vi "运维调试_CODCr.vi"() -> ()   [LabVIEW 2016, in "CODCr库.lvlib"]
uses:
  <vilib>/Utility/miscctls.llb/LVPointTypeDef.ctl
  <vilib>/ptbypt/NI_PtbyPt.lvlib
  <vilib>/Utility/config.llb/NI_LVConfig.lvlib
panel:
  in  "质控参数":bool
  in  "仪器参数":bool
  in  "MB通信方式选择":enum16{"串口", "TCP"}(ring)
  in  "释放串口":bool
  in  "打开串口":bool
  in  "加标回收测试":bool
  in  "平行样测试":bool
  in  "定时启动":bool
  out "COM口":string
  in  "空白测试":bool
  in  "隐藏按钮":bool
  in  "写入消解温度时长":bool
  in  "保存KB值":bool
  in  "标样核查":bool
  out "启动时间":timestamp format="%<%Y/%m/%d %H:%M:%S>T"
  out "主循环次数":i32
  out "status":bool
  out "启动测量模式":T1(ring)
  out "曲线截距B":sgl format="%#_10g"
  out "曲线斜率K":sgl format="%#_10g"
  out "量程上限":sgl
  out "量程下限":sgl
  out "消解时长":u16
  out "消解温度":u16
  out "测量精度":u16
  out "测量结果":sgl
  out "标样参考值":sgl
  out "量程":u16
  out "工作状态":T1(ring)
  out "仪器时间":timestamp format="%<%X\n%x>T"
  out "关键参数区":T2
  out "状态告警区":T3 {"告警代码" items=["无告警", "缺试剂告警", "缺水样告警", "缺蒸馏水告警", "缺标液告警", "仪表漏液告警", "标定异常告警", "超量程告警", "加热异常", "低试剂预警", "超上限告警", "超下限告警", "仪表内部其他异常", "滴定异常告警", "电极异常告警", "量程切换告警", "参数设置告警", "PH电极电位异常", "电导率电极异常", "浊度光度异常", "溶解氧电极异常", "溶解氧光强异常", "温度异常告警", "PH异常告警", "溶解氧异常告警", "电导率异常告警", "浊度异常告警", "叶绿素异常告警", "藻密度异常告警", "蓝绿藻异常告警", "ORP异常告警", "氨氮异常告警", "清洁刷异常告警", "SD卡异常告警", "蓝牙异常告警", "Wifi异常告警", "流程异常告警"]; "故障代码" items=["无故障", "电机故障", "温度故障", "通讯故障", "滴定故障"]}
  out "测量数据区":T4 {"单位" items=["ug/L", "mg/L", "ppm", "mg/m3", "cm", "ppb", "ug/m3", "%", "nmol/mol", "umol/mol", "MPN/L", "MPN/100ml", "ng/m3", "NTU", "无量纲", "ms/cm", "us/cm", "℃", "mV", "万个/L"]}
  out "系统时间":timestamp format="%<%Y/%m/%d %H:%M:%S>T"
  in  "停止":bool
  in  "校时":bool
  in  "标样校准":bool
  in  "空白校准":bool
  in  "零点核查":bool
  in  "跨度核查":bool
  in  "水样测试":bool
  in  "返回":bool
  in  "设置":bool
  # "mg/L"
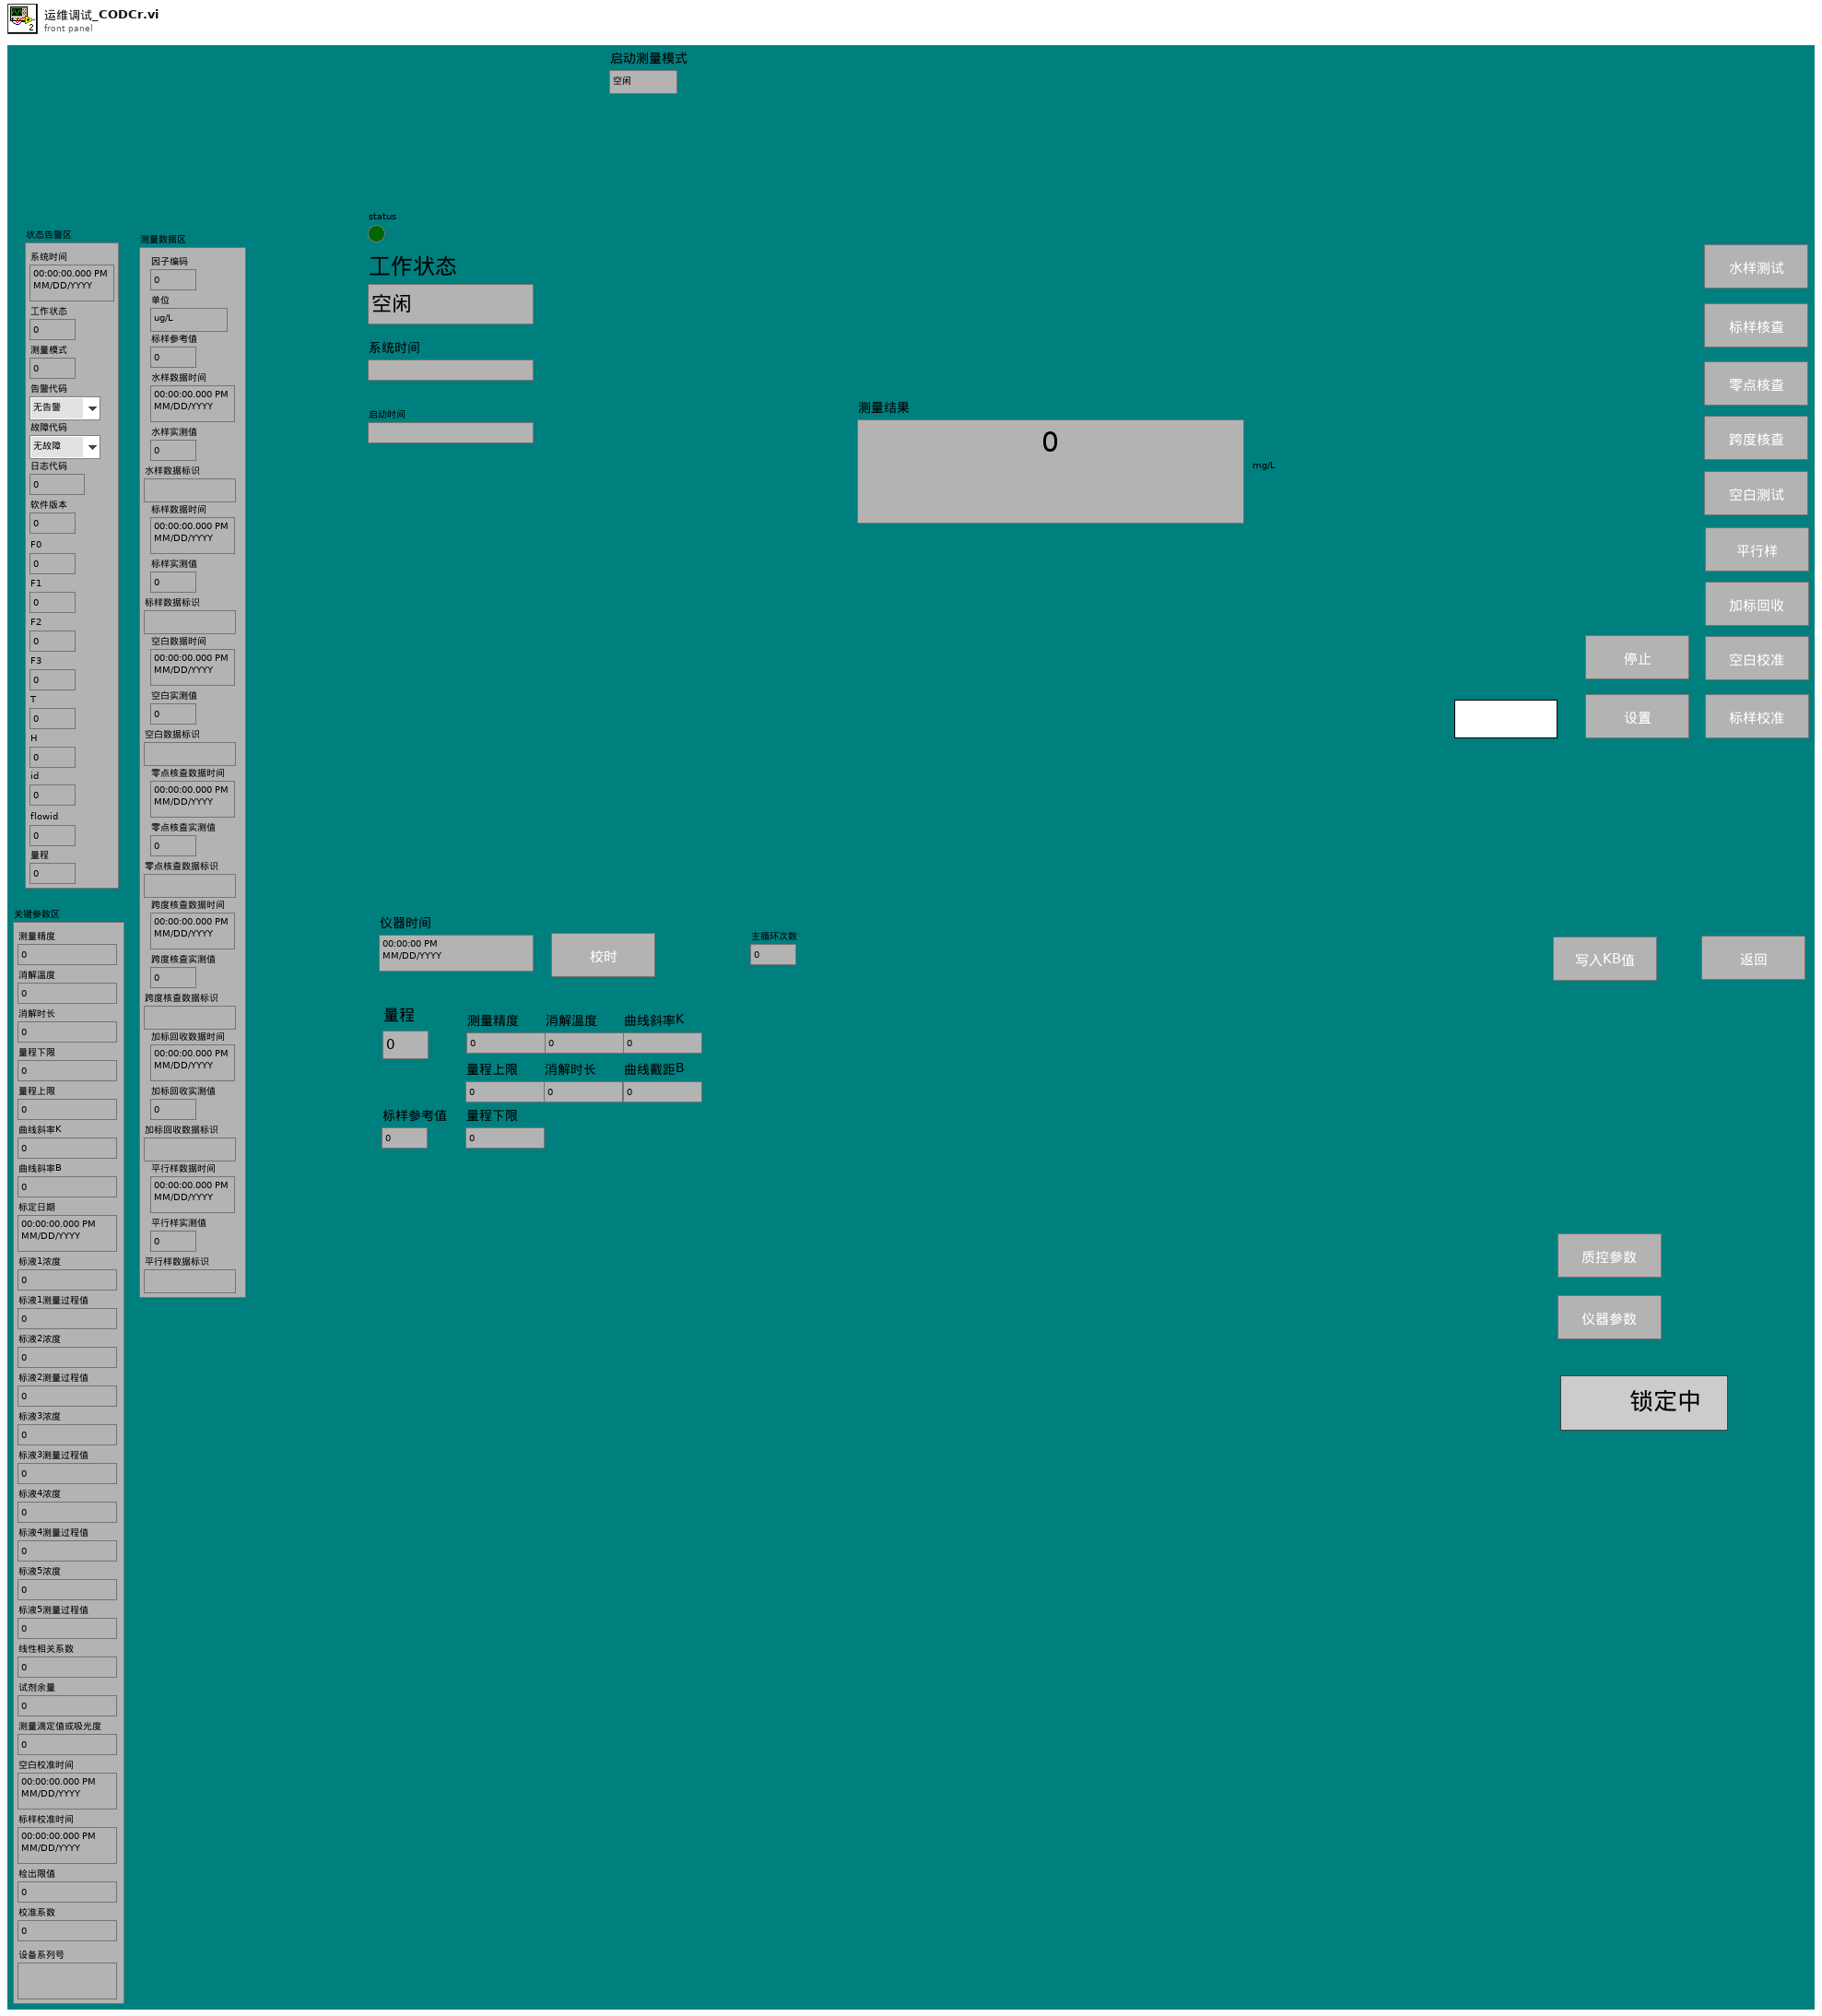
[diagram p1: front panel]
types:
  T1 = enum16{"空闲", "水样测试", "标样核查", "零点核查", "跨度核查", "空白测试", "平行样测试", "加标回收", "空白校准", "标样校准", "初始化（清洗）"}
  T2 = cluster{"测量精度":u16, "消解温度":u16, "消解时长":u16, "量程下限":sgl, "量程上限":sgl, "曲线斜率K":sgl, "曲线斜率B":sgl, "标定日期":timestamp, "标液1浓度":sgl, "标液1测量过程值":sgl, "标液2浓度":sgl, "标液2测量过程值":sgl, "标液3浓度":sgl, "标液3测量过程值":sgl, "标液4浓度":sgl, "标液4测量过程值":sgl, "标液5浓度":sgl, "标液5测量过程值":sgl, "线性相关系数":sgl, "试剂余量":u32, "测量滴定值或吸光度":sgl, "空白校准时间":timestamp, "标样校准时间":timestamp, "检出限值":sgl, "校准系数":sgl, "设备系列号":string}
  T3 = cluster{"系统时间":timestamp, "工作状态":u16, "测量模式":u16, "告警代码":u16, "故障代码":u16, "日志代码":u16, "软件版本":u16, "F0":sgl, "F1":sgl, "F2":sgl, "F3":sgl, "T":sgl, "H":sgl, "id":u16, "flowid":u16, "量程":u16}
  T4 = cluster{"因子编码":u32, "单位":u16, "标样参考值":sgl, "水样数据时间":timestamp, "水样实测值":sgl, "水样数据标识":string, "标样数据时间":timestamp, "标样实测值":sgl, "标样数据标识":string, "空白数据时间":timestamp, "空白实测值":sgl, "空白数据标识":string, "零点核查数据时间":timestamp, "零点核查实测值":sgl, "零点核查数据标识":string, "跨度核查数据时间":timestamp, "跨度核查实测值":sgl, "跨度核查数据标识":string, "加标回收数据时间":timestamp, "加标回收实测值":sgl, "加标回收数据标识":string, "平行样数据时间":timestamp, "平行样实测值":sgl, "平行样数据标识":string}
  T5 = cluster{"命令":string, "测量模式":enum16{"水样测量", "标样核查", "零点核查", "跨度核查", "空白测试", "加标回收", "平行样", "校零", "校标"}, "CODCr量程切换":enum32{"H", "L", "AUTO"}}
  T6 = typedef "LVPointTypeDef.ctl" = cluster{"Horizontal":i16, "Vertical":i16}
  T7 = typedef "NI_LVConfig.lvlib/Config Data RefNum.ctl" = refnum<k1>
  T8 = cluster{"运行模式":enum16{"维护模式", "常规模式", "应急模式", "质控模式"}}
  T9 = cluster{"时间标识":timestamp, "监测值":sgl, "单位":u16, "数据标识":string, "因子编码":u32, "标样参考值":sgl, "F0":sgl, "F1":sgl, "F2":sgl, "F3":sgl, "温度":sgl, "湿度":sgl, "量程标识":string, "LastTime":timestamp}
  T10 = cluster{"时间标识":timestamp, "设备":string, "日志信息":string}
  T11 = cluster{"时间标识":timestamp, "参数":string, "日志信息":string, "流程参数":string}
  T12 = cluster{"时间标识":timestamp, "设备":string, "日志信息":string, "流程参数":string}
  T13 = enum16{"水样测量", "标样核查", "零点核查", "跨度核查", "空白测试", "加标回收", "平行样", "校零", "校标"}
  T14 = cluster{"控制命令":enum16{"启动测量", "标样核查", "零点核查", "跨度核查", "空白测试", "平行样测试", "加标回收", "空白校准", "标样校准", "初始化（清洗）", "停止测试", "仪器重启", "校时", "模式设置", "测量间隔设置"}, "周期设置类型":enum16{"定点启动", "间隔启动"}, "定时功能启用":bool, "定时间隔":dbl, "24H周期设置":bool[], "零点核查时间":u16, "跨度核查时间":u16, "质控频次":enum16{"关闭", "每天", "星期一", "星期二", "星期三", "星期四", "星期五", "星期六", "星期日"}}
  T15 = cluster{"测量量程":dbl, "测量精度":dbl, "测量间隔":dbl, "消解温度":dbl, "消解时长":dbl, "空白校准时间":timestamp, "曲线截距":dbl, "曲线斜率":dbl, "测量检出限":dbl, "测量信号值":dbl, "线性相关系数":dbl, "二次多项式系数":dbl, "标样校准时间":timestamp, "稀释倍数":dbl, "三项式系数":dbl, "空白标定系数":dbl, "量程系数":dbl, "F0/ORPA":dbl, "F1/ORPB":dbl, "F2/ORPK":dbl, "F3":dbl, "F4":dbl, "F5":dbl, "F6":dbl, "F7":dbl, "X0/滴定数":dbl, "量程":dbl}
  T16 = cluster{"控制命令":enum16{"启动测量", "标样核查", "零点核查", "跨度核查", "空白测试", "平行样测试", "加标回收", "空白校准", "标样校准", "初始化（清洗）", "停止测试", "仪器重启", "校时", "模式设置", "测量间隔设置"}, "周期设置类型":enum16{"定点启动", "间隔启动"}, "定时功能启用":bool, "定时间隔":dbl, "24H周期设置":bool[], "空白核查时间":u16, "跨度核查时间":u16, "质控频次":enum16{"关闭", "每天", "星期一", "星期二", "星期三", "星期四", "星期五", "星期六", "星期日"}}
  T17 = cluster{"确定":bool, "测量量程":dbl, "测量精度":dbl, "测量间隔":dbl, "消解温度":dbl, "消解时长":dbl, "空白校准时间":timestamp, "曲线截距":dbl, "曲线斜率":dbl, "测量检出限":dbl, "测量信号值":dbl, "线性相关系数":dbl, "二次多项式系数":dbl, "标样校准时间":timestamp, "稀释倍数":dbl, "三项式系数":dbl, "空白标定系数":dbl, "量程系数":dbl, "F0/ORPA":dbl, "F1/ORPB":dbl, "F2/ORPK":dbl, "F3":dbl, "F4":dbl, "F5":dbl, "F6":dbl, "F7":dbl, "X0/滴定数":dbl, "量程":dbl}
  T18 = cluster{"跨度值":dbl, "零点标准液浓度":dbl, "跨度标准液浓度":dbl, "标准液标准浓度":dbl}
  T19 = cluster{"确定":bool, "跨度值":dbl, "零点标准液浓度":dbl, "跨度标准液浓度":dbl, "标准液标准浓度":dbl}
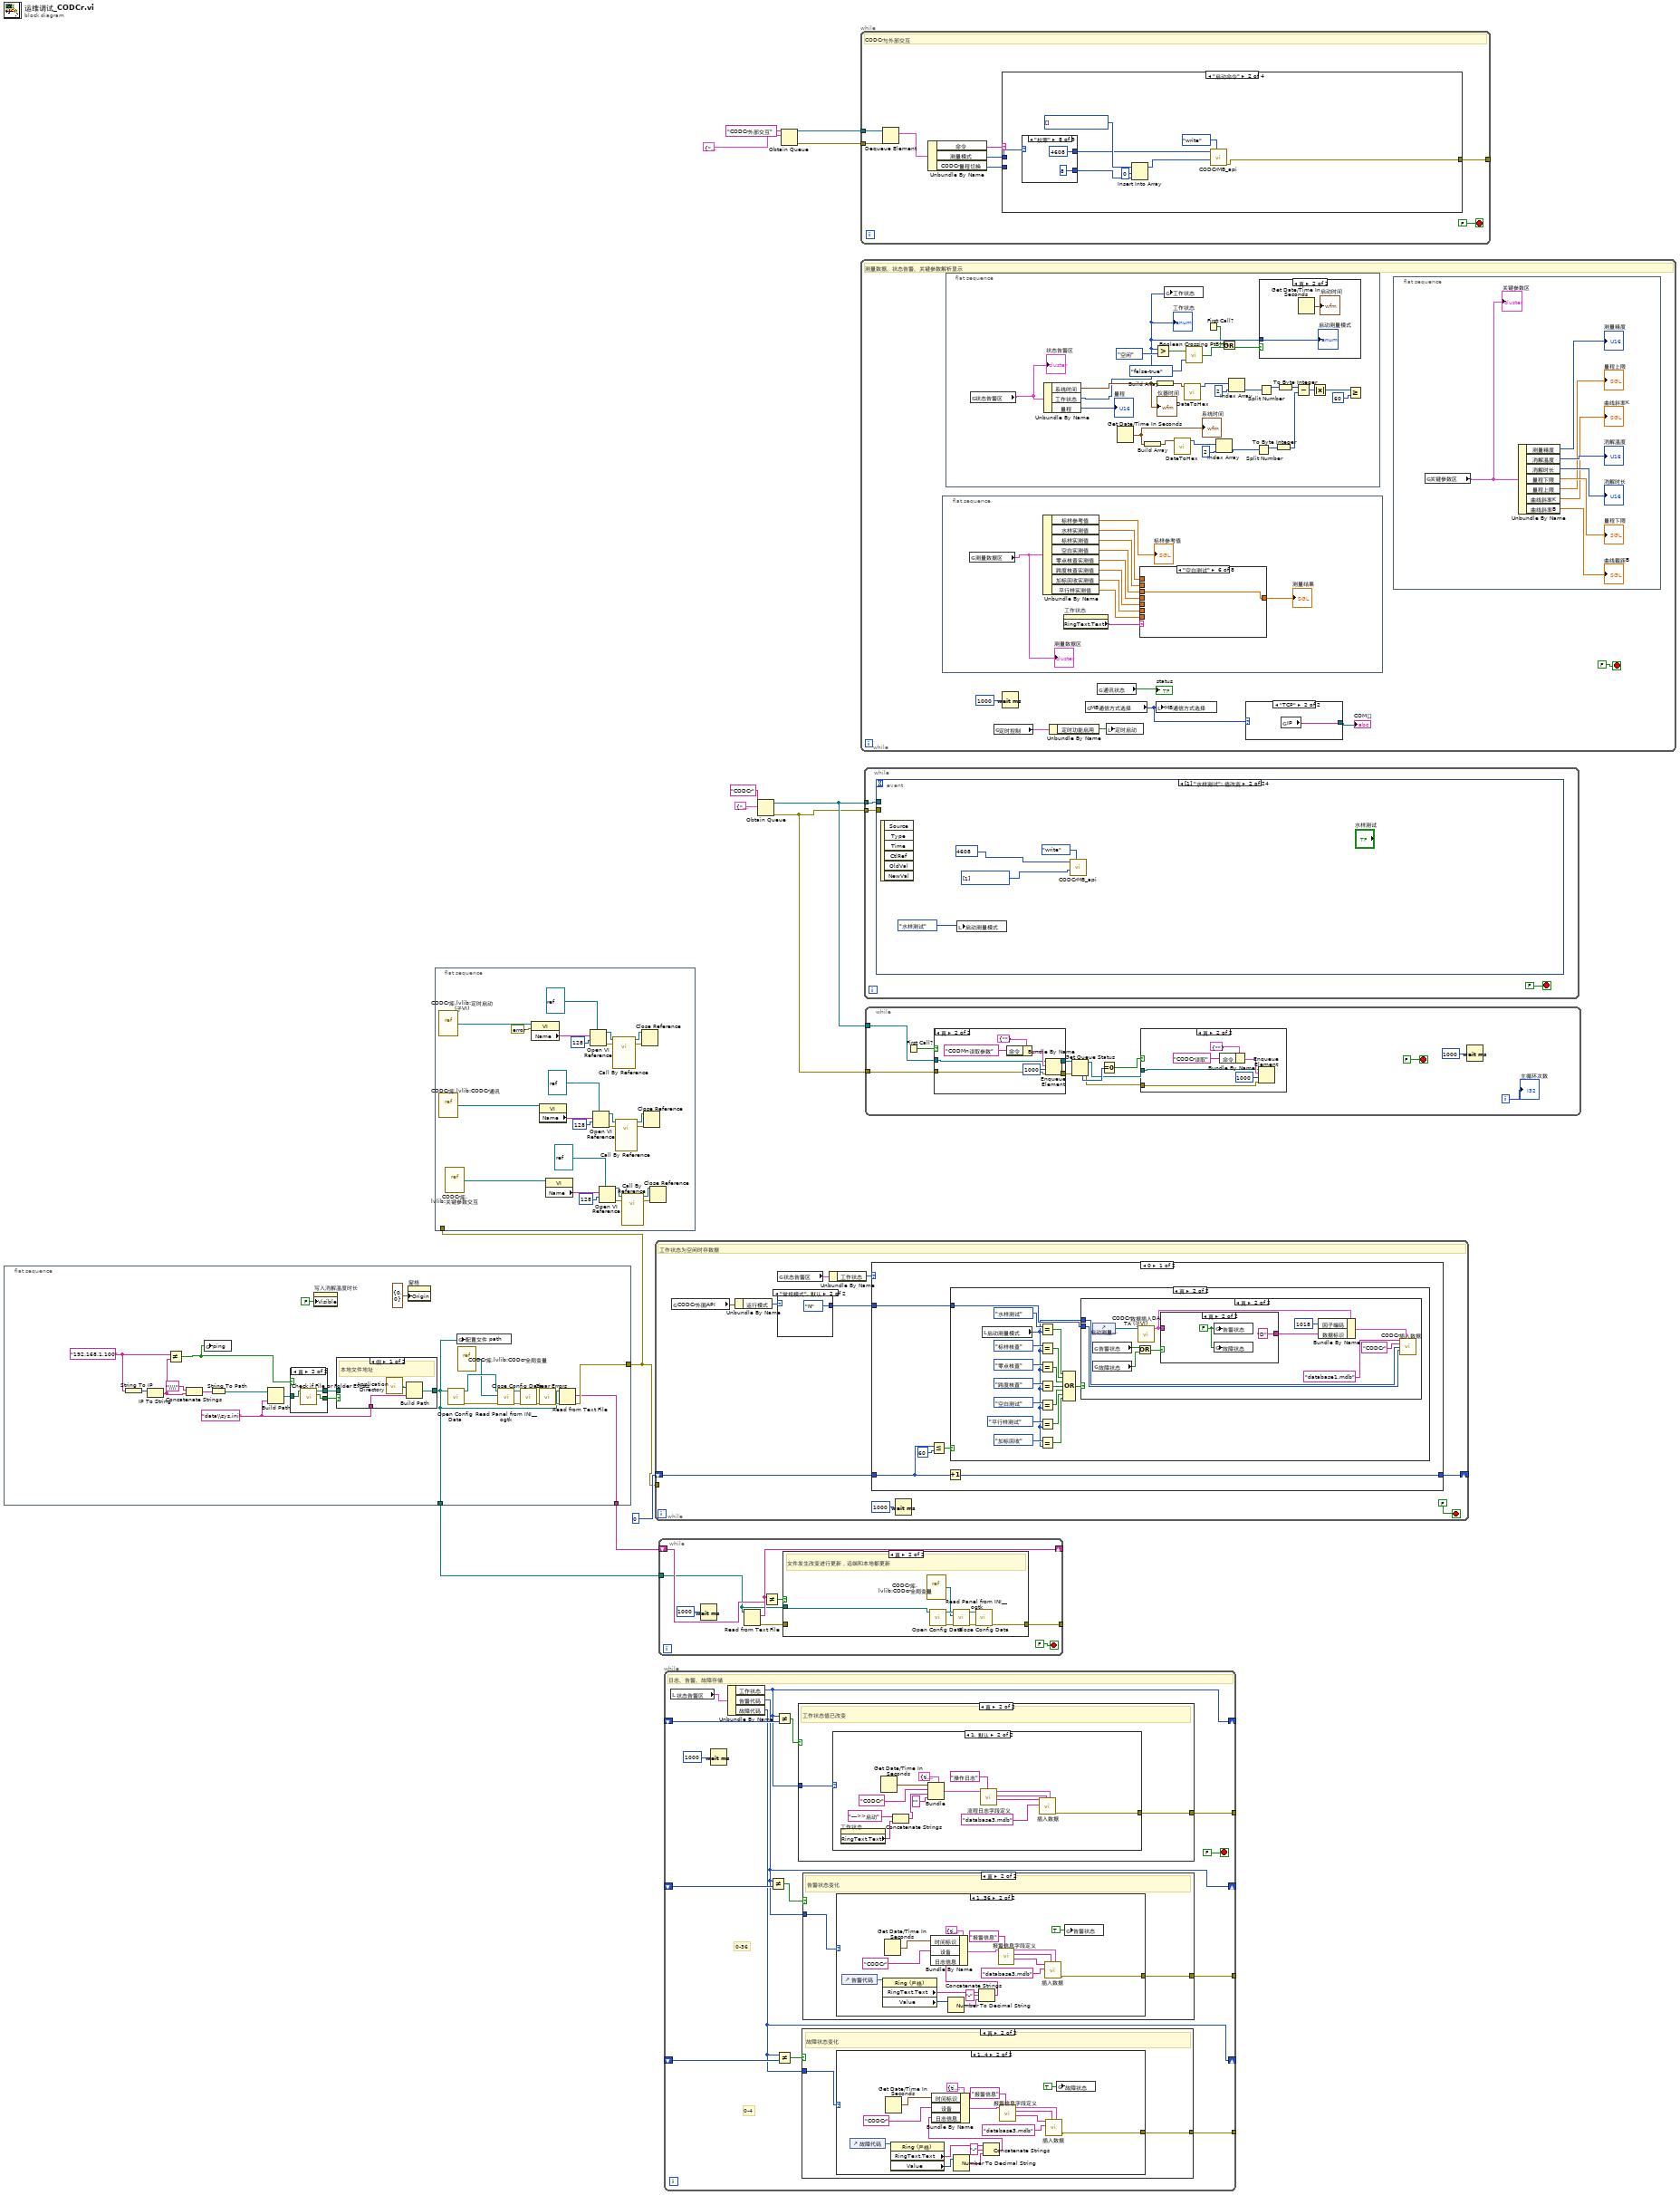
[diagram p0: block diagram]
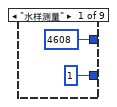
[diagram p6: hidden frame]
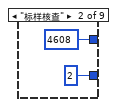
[diagram p7: hidden frame]
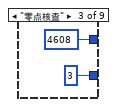
[diagram p8: hidden frame]
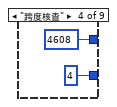
[diagram p9: hidden frame]
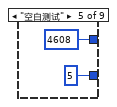
[diagram p10: hidden frame]
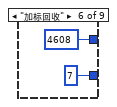
[diagram p11: hidden frame]
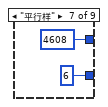
[diagram p12: hidden frame]
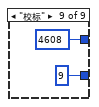
[diagram p13: hidden frame]
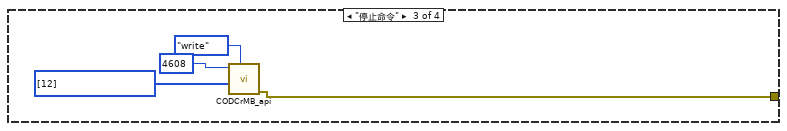
[diagram p14: hidden frame]
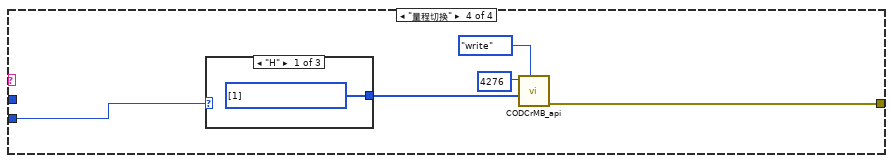
[diagram p15: hidden frame]
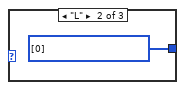
[diagram p16: hidden frame]
diagram:
  n1 = flat-sequence {
    tunnel: [w15] -> w1
    tunnel: [w14] -> w3
    tunnel: [w13] -> w2
    frame #0 {
      w33 = "data\\sys.ini" ("名称或相对路径")
      w18 = "192.168.1.100" ("名称")
      n2 = String To IP(1:w18) -> (0:w25:u32)
      n3 = IP To String(2:w25) -> (0:w22:string)  [unwired: 1 in]
      n4 = Not Equal?(x=w18, y=w22) -> (x != y?=w32:bool)
      n5 = Concatenate Strings("\\\\" ("字符串"), w22) -> (w23:string)
      n6 = global write "CODcr全局变量.vi" "ping"(w32) -> ()
      n7 = String To Path(string=w23) -> (path=w17:path)
      n8 = Build Path(base path=w17, name or relative path=w33) -> (appended path=w21:path)
      n9 = case shown="真" w32 {
        tunnel: w21 -> [w36 w40]
        tunnel: [w36 w39] -> w20
        tunnel: [FALSE w38] -> w19
        frame False {
        }
        frame True {
          n10 = call <vilib>:"Check if File or Folder Exists.vi"("path"=w40) -> ("file or folder exists?"=w38:bool, "dup path"=w39:path)  [unwired: 8 in, 1 out]
        }
      }
      n11 = property on="写入消解温度时长" class="Bool"("Visible"=FALSE ("可见")) -> ()  [unwired: 2 in, 2 out]
      n12 = case shown="假" w19 {
        tunnel: w20 -> [_ w44]
        tunnel: [w42 w44] -> w13
        tunnel: w33 -> [w41 _]
        frame False {
          # "本地文件地址"
          n13 = call <vilib>:"Application Directory.vi"() -> ("Application Directory"=w43:path)
          n14 = Build Path(base path=w43, name or relative path=w41) -> (appended path=w42:path)
        }
        frame True {
          # "网络共享地址"
        }
      }
      n15 = property on="窗格" class="Pane"("Origin"=T6 {"Horizontal"=0, "Vertical"=0} ("原点")) -> ()  [unwired: 2 in, 2 out]
      n16 = call <vilib>:"Open Config Data.vi"("configuration file path"=w13) -> ("error out"=w29:errorcluster, "refnum"=w28:T7)  [unwired: 8 in, 1 out]
      n17 = global write "CODcr全局变量.vi" "配置文件 path"(w13) -> ()
      n18 = vi-ref "CODCr库.lvlib:CODcr全局变量.vi"() -> (w16:refnum<vi>)
      n19 = call <userlib>:"Read Panel from INI__ogtk.vi"("error in (no error)"=w29, "VI ref"=w16, "refnum"=w28) -> ("error out"=w27:errorcluster, "refnum out"=w26:T7)  [unwired: 7 in]
      n20 = call <vilib>:"Close Config Data.vi"("error in (no error)"=w27, "refnum"=w26) -> ("error out"=w30:errorcluster)  [unwired: 8 in, 1 out]
      n21 = call <vilib>:"Clear Errors.vi"("error in (no error)"=w30) -> ("error out"=w31:errorcluster)  [unwired: 5 in, 1 out]
      n22 = Read from Text File(file (use dialog)=w13, error in=w31) -> (text=w14:string, error out=w15:errorcluster)  [unwired: 2 in, 2 out]
    }
  }
  n23 = flat-sequence {
    tunnel: w1 -> [_]
    frame #0 {
      n24 = vi-ref "CODCr库.lvlib:定时启动 (子VI).vi"() -> (w53:refnum<vi>)
      n25 = vi-ref "CODCr库.lvlib:CODCr通讯.vi"() -> (w62:refnum<vi>)
      n26 = vi-ref "CODCr库.lvlib:关键参数交互.vi"() -> (w52:refnum<vi>)
      n27 = property class="VI"(reference=w53, error in=errorcluster {"status"=FALSE, "code"=0, "source"=""} ("错误输出")) -> ("Name"=w54:string)  [unwired: 2 out]
      n28 = property class="VI"(reference=w62) -> ("Name"=w63:string)  [unwired: 1 in, 2 out]
      n29 = property class="VI"(reference=w52) -> ("Name"=w51:string)  [unwired: 1 in, 2 out]
      n30 = Open VI Reference(type specifier VI Refnum (for type only)=refnum<vi> refnum, vi path=w54, options=128 ("选项")) -> (vi reference=w56:refnum<vi>, error out=w58:errorcluster)  [unwired: 3 in]
      n31 = Open VI Reference(type specifier VI Refnum (for type only)=refnum<vi> refnum, vi path=w63, options=128 ("选项")) -> (vi reference=w65:refnum<vi>, error out=w67:errorcluster)  [unwired: 3 in]
      n32 = Open VI Reference(type specifier VI Refnum (for type only)=refnum<vi> refnum, vi path=w51, options=128 ("选项")) -> (vi reference=w49:refnum<vi>, error out=w47:errorcluster)  [unwired: 3 in]
      n33 = call-by-ref "?"(reference=w56, error in=w58) -> (reference out=w60:refnum<vi>, error out=w59:errorcluster)  [unwired: 12 in]
      n34 = call-by-ref "?"(reference=w65, error in=w67) -> (reference out=w69:refnum<vi>, error out=w68:errorcluster)  [unwired: 12 in]
      n35 = call-by-ref "?"(reference=w49, error in=w47) -> (reference out=w45:refnum<vi>, error out=w46:errorcluster)  [unwired: 12 in]
      n36 = Close Reference(reference=w60, error in (no error)=w59) -> ()  [unwired: 1 out]
      n37 = Close Reference(reference=w69, error in (no error)=w68) -> ()  [unwired: 1 out]
      n38 = Close Reference(reference=w45, error in (no error)=w46) -> ()  [unwired: 1 out]
    }
  }
  n39 = while "While循环" {
    tunnel: w1 -> [_]
    shift-right: [w70] -> _
    shift-left: 0 -> [w71]
    stop <- FALSE stop-if-true
    # "工作状态为空闲时存数据"
    n40 = global read "CODCr外部API.vi" "CODCr外围API"() -> (w74:T8)
    n41 = Unbundle By Name(w74) -> ("运行模式"=w73:enum16{"维护模式", "常规模式", "应急模式", "质控模式"})
    n42 = global read "CODcr全局变量.vi" "状态告警区"() -> (w72:T3)
    n43 = case shown="\"常规模式\", 默认" w73 {
      tunnel: [enum16{"N", "M"}."M" ("数据类型") enum16{"N", "M"}."N" ("数据类型")] -> w75
      frame "维护模式" {
      }
      frame "常规模式", Default {
      }
    }
    n44 = Unbundle By Name(w72) -> ("工作状态"=w76:u16)
    n45 = case shown="0" w76 {
      tunnel: w75 -> [w85 _]
      tunnel: w71 -> [w83 _]
      tunnel: [w84 _] -> w70
      frame 0 {
        n46 = Less Or Equal?(x=w83, y=60) -> (x <= y?=w81:bool)
        n47 = Increment(x=w83) -> (x+1=w84:i32)
        n48 = case shown="真" w81 {
          tunnel: w85 -> [_ w102]
          frame False {
          }
          frame True {
            n49 = local read "启动测量模式"() -> (w94:T1)
            n50 = Equal?(x=T1."水样测试" ("启动测量模式"), y=w94) -> (x = y?=w93:bool)
            n51 = Equal?(x=T1."标样核查" ("启动测量模式"), y=w94) -> (x = y?=w92:bool)
            n52 = Equal?(x=T1."零点核查" ("启动测量模式"), y=w94) -> (x = y?=w91:bool)
            n53 = Equal?(x=T1."跨度核查" ("启动测量模式"), y=w94) -> (x = y?=w90:bool)
            n54 = Equal?(x=T1."空白测试" ("启动测量模式"), y=w94) -> (x = y?=w89:bool)
            n55 = Equal?(x=T1."平行样测试" ("启动测量模式"), y=w94) -> (x = y?=w88:bool)
            n56 = Equal?(x=T1."加标回收" ("启动测量模式"), y=w94) -> (x = y?=w87:bool)
            n57 = Compound Arithmetic op=OR(w93, w92, w91, w90, w89, w88, w87) -> (w86:bool)
            n58 = case shown="真" w86 {
              tunnel: w94 -> [_ w110]
              tunnel: w102 -> [_ w109]
              frame False {
              }
              frame True {
                n59 = control-ref of="启动测量模式"() -> (w114:refnum<vi>)
                n60 = global read "CODcr全局变量.vi" "告警状态"() -> (w107:bool)
                n61 = global read "CODcr全局变量.vi" "故障状态"() -> (w106:bool)
                n62 = Or(x=w107, y=w106) -> (x .or. y?=w105:bool)
                n63 = call "CODCr数据插入DATA (子VI).vi"("Enum输入"=w114) -> ("data"=w104:T9)  [unwired: 10 in]
                n64 = case shown="真" w105 {
                  tunnel: w104 -> [w116 _]
                  tunnel: [w115 "D" ("table")] -> w103
                  frame False {
                    n65 = Unbundle By Name(w116) -> ("数据标识"=w115:string)
                  }
                  frame True {
                    w117 = FALSE ("告警状态")
                    n66 = global write "CODcr全局变量.vi" "告警状态"(w117) -> ()
                    n67 = global write "CODcr全局变量.vi" "故障状态"(w117) -> ()
                  }
                }
                n68 = Bundle By Name(cluster=w104, "因子编码"=u32 1018, "数据标识"=w103) -> (w113:T9)
                n69 = call "CODCr插入数据.vi"("database"="database1.mdb", "data"=w113, "table"="CODCr", "测量模式"=w110, "数据类型"=w109) -> ()  [unwired: 10 in, 1 out]
              }
            }
          }
        }
      }
      frame 1, Default {
      }
    }
    n70 = Wait (ms)(milliseconds to wait=u32 1000 ("等待时间（毫秒）")) -> ()  [unwired: 1 out]
  }
  n71 = while {
    tunnel: [w125] -> _
    shift-right: [w123] -> _
    shift-left: w3 -> [w122]
    tunnel: w2 -> [w119]
    stop <- FALSE stop-if-true
    n72 = Wait (ms)(milliseconds to wait=u32 1000 ("等待时间（毫秒）")) -> ()  [unwired: 1 out]
    n73 = Read from Text File(file (use dialog)=w119) -> (text=w123:string, error out=w120:errorcluster)  [unwired: 3 in, 2 out]
    n74 = Not Equal?(x=w123, y=w122) -> (x != y?=w121:bool)
    n75 = case shown="真" w121 {
      tunnel: [w127 w134] -> w125
      tunnel: w119 -> [_ w128]
      tunnel: w120 -> [w127 _]
      frame False {
      }
      frame True {
        # "文件发生改变进行更新，远端和本地都更新"
        n76 = vi-ref "CODCr库.lvlib:CODcr全局变量.vi"() -> (w129:refnum<vi>)
        n77 = call <vilib>:"Open Config Data.vi"("configuration file path"=w128) -> ("error out"=w133:errorcluster, "refnum"=w132:T7)  [unwired: 8 in, 1 out]
        n78 = call <userlib>:"Read Panel from INI__ogtk.vi"("error in (no error)"=w133, "VI ref"=w129, "refnum"=w132) -> ("error out"=w131:errorcluster, "refnum out"=w130:T7)  [unwired: 7 in]
        n79 = call <vilib>:"Close Config Data.vi"("error in (no error)"=w131, "refnum"=w130) -> ("error out"=w134:errorcluster)  [unwired: 8 in, 1 out]
      }
    }
  }
  n80 = while {
    shift-right: [w145] -> _
    shift-left: _ -> [w147]
    tunnel: [w144] -> _
    shift-right: [w141] -> _
    shift-left: _ -> [w142]
    shift-right: [w137] -> _
    shift-left: _ -> [w139]
    tunnel: [w138] -> _
    tunnel: [w136] -> _
    stop <- FALSE stop-if-true
    # "0-4"
    # "0-36"
    # "日志、告警、故障存储"
    n81 = local read "状态告警区"() -> (w135:T3)
    n82 = Wait (ms)(milliseconds to wait=u32 1000 ("等待时间（毫秒）")) -> ()  [unwired: 1 out]
    n83 = Unbundle By Name(w135) -> ("工作状态"=w145:u16, "告警代码"=w141:u16, "故障代码"=w137:u16)
    n84 = Not Equal?(x=w141, y=w142) -> (x != y?=w143:bool)
    n85 = Not Equal?(x=w145, y=w147) -> (x != y?=w146:bool)
    n86 = Not Equal?(x=w137, y=w139) -> (x != y?=w140:bool)
    n87 = case shown="真" w146 {
      tunnel: w145 -> [_ w189]
      tunnel: [_ w188] -> w144
      frame False {
      }
      frame True {
        # "工作状态值已改变"
        n88 = case shown="1, 默认" w189 {
          tunnel: [w190 w205] -> w188
          frame 0 {
            n89 = Get Date/Time In Seconds() -> (seconds since 1Jan1904=w197:timestamp)
            n90 = Bundle(cluster=T11 {"时间标识"=timestamp(0 s since 1904-01-01), "参数"="", "日志信息"="", "流程参数"=""} ("data in"), "时间标识"=w197, "参数"="CODCr" ("table输入"), "日志信息"="--->>结束", "流程参数"="" ("table输入")) -> (w191:T11)
            n91 = call "流程日志字段定义.vi"("table输入"="操作日志", "data in"=w191) -> ("table输出"=w195:string, "columns"=w193:string[], "data out"=w192:T12)  [unwired: 7 in]
            n92 = call "插入数据.vi"("data"=w192, "columns"=w193, "database"="database3.mdb", "table"=w195) -> ("error out"=w190:errorcluster)  [unwired: 7 in]
          }
          frame 1, Default {
            n93 = property on="工作状态" class="Enum (严格)"() -> ("RingText.Text"=w202:string)  [unwired: 2 in, 2 out]
            n94 = Get Date/Time In Seconds() -> (seconds since 1Jan1904=w212:timestamp)
            n95 = Concatenate Strings("--->>启动" ("日志信息"), w202) -> (w203:string)
            n96 = Bundle(cluster=T11 {"时间标识"=timestamp(0 s since 1904-01-01), "参数"="", "日志信息"="", "流程参数"=""} ("data in"), "时间标识"=w212, "参数"="CODCr" ("table输入"), "日志信息"=w203, "流程参数"="" ("table输入")) -> (w211:T11)
            n97 = call "流程日志字段定义.vi"("table输入"="操作日志", "data in"=w211) -> ("table输出"=w209:string, "columns"=w207:string[], "data out"=w206:T12)  [unwired: 7 in]
            n98 = call "插入数据.vi"("data"=w206, "columns"=w207, "database"="database3.mdb", "table"=w209) -> ("error out"=w205:errorcluster)  [unwired: 7 in]
          }
        }
      }
    }
    n99 = case shown="真" w140 {
      tunnel: w137 -> [_ w151]
      tunnel: [_ w150] -> w136
      frame False {
      }
      frame True {
        # "故障状态变化"
        n100 = case shown="1..4" w151 {
          tunnel: [_ w158] -> w150
          frame 0, Default {
            # "无告警"
          }
          frame 1..4 {
            n101 = control-ref of="故障代码"() -> (w168:refnum<vi>)
            n102 = Get Date/Time In Seconds() -> (seconds since 1Jan1904=w166:timestamp)
            n103 = property class="Ring (严格)"(reference=w168) -> ("RingText.Text"=w155:string, "Value"=w156:u16)  [unwired: 1 in, 2 out]
            n104 = Number To Decimal String(number=w156) -> (decimal integer string=w153:string)  [unwired: 1 in]
            n105 = Concatenate Strings(w155, "-" ("字符串"), w153) -> (w154:string)
            n106 = Bundle By Name(cluster=T10 {"时间标识"=timestamp(0 s since 1904-01-01), "设备"="", "日志信息"=""} ("data in"), "时间标识"=w166, "设备"="CODCr" ("table输入"), "日志信息"=w154) -> (w165:T10)
            n107 = call "报警信息字段定义.vi"("table输入"="报警信息", "data in"=w165) -> ("table输出"=w160:string, "columns"=w159:string[], "data out"=w162:T10)  [unwired: 7 in]
            n108 = call "插入数据.vi"("data"=w162, "columns"=w159, "database"="database3.mdb", "table"=w160) -> ("error out"=w158:errorcluster)  [unwired: 7 in]
            n109 = global write "CODcr全局变量.vi" "故障状态"(TRUE ("告警状态")) -> ()
          }
        }
      }
    }
    n110 = case shown="真" w143 {
      tunnel: w141 -> [_ w170]
      tunnel: [_ w169] -> w138
      frame False {
      }
      frame True {
        # "告警状态变化"
        n111 = case shown="1..36" w170 {
          tunnel: [_ w180] -> w169
          frame 0, Default {
            # "无告警"
          }
          frame 1..36 {
            n112 = control-ref of="告警代码"() -> (w177:refnum<vi>)
            n113 = property class="Ring (严格)"(reference=w177) -> ("RingText.Text"=w175:string, "Value"=w174:u16)  [unwired: 1 in, 2 out]
            n114 = Get Date/Time In Seconds() -> (seconds since 1Jan1904=w179:timestamp)
            n115 = Number To Decimal String(number=w174) -> (decimal integer string=w171:string)  [unwired: 1 in]
            n116 = Concatenate Strings(w175, "-" ("字符串"), w171) -> (w173:string)
            n117 = Bundle By Name(cluster=T10 {"时间标识"=timestamp(0 s since 1904-01-01), "设备"="", "日志信息"=""} ("data in"), "时间标识"=w179, "设备"="CODCr" ("table输入"), "日志信息"=w173) -> (w181:T10)
            n118 = call "报警信息字段定义.vi"("table输入"="报警信息", "data in"=w181) -> ("table输出"=w186:string, "columns"=w187:string[], "data out"=w184:T10)  [unwired: 7 in]
            n119 = call "插入数据.vi"("data"=w184, "columns"=w187, "database"="database3.mdb", "table"=w186) -> ("error out"=w180:errorcluster)  [unwired: 7 in]
            n120 = global write "CODcr全局变量.vi" "告警状态"(TRUE ("告警状态")) -> ()
          }
        }
      }
    }
  }
  n121 = Obtain Queue(name (unnamed)="CODCr" ("名称（未命名）"), element data type=cluster{"命令":string} {"命令"="启用模块"} ("元素")) -> (queue out=w6:refnum<queue>, error out=w5:errorcluster)  [unwired: 3 in, 1 out]
  n122 = Obtain Queue(name (unnamed)="CODCr外部交互" ("名称（未命名）"), element data type=T5 {"命令"="启动命令", "测量模式"=enum."水样测量", "CODCr量程切换"=enum."AUTO"} ("元素")) -> (queue out=w8:refnum<queue>, error out=w7:errorcluster)  [unwired: 3 in, 1 out]
  n123 = while {
    tunnel: w8 -> [w221]
    tunnel: w7 -> [w220]
    tunnel: [w216] -> _
    stop <- FALSE stop-if-true
    # "CODCr与外部交互"
    n124 = Dequeue Element(queue=w221, error in (no error)=w220) -> (element=w222:T5)  [unwired: 1 in, 3 out]
    n125 = Unbundle By Name(w222) -> ("命令"=w219:string, "测量模式"=w218:T13, "CODCr量程切换"=w217:enum32{"H", "L", "AUTO"})
    n126 = case shown="\"启动命令\"" w219 {
      tunnel: w218 -> [_ w225 _ _]
      tunnel: w217 -> [_ _ _ w255]
      tunnel: [_ w224 w250 w254] -> w216
      frame "假", Default {
      }
      frame "启动命令" {
        n127 = case shown="\"校零\"" w225 {
          tunnel: [u16 4608 ("address") u16 4608 ("address") u16 4608 ("address") u16 4608 ("address") u16 4608 ("address") u16 4608 ("address") u16 4608 ("address") u16 4608 ("address") u16 4608 ("address")] -> w227
          tunnel: [u16 1 ("address") u16 2 ("address") u16 3 ("address") u16 4 ("address") u16 5 ("address") u16 7 ("address") u16 6 ("address") u16 8 ("address") u16 9 ("address")] -> w231
          frame "水样测量" {
          }
          frame "标样核查" {
          }
          frame "零点核查" {
          }
          frame "跨度核查" {
          }
          frame "空白测试" {
          }
          frame "加标回收" {
          }
          frame "平行样" {
          }
          frame "校零" {
          }
          frame "校标" {
          }
        }
        n128 = Insert Into Array(array=u16[] [] ("values"), index=0 ("索引"), new element=w231) -> (w226:u16[])
        n129 = call "CODCrMB_api.vi"("STEP"=enum16{"open", "read", "write", "close"}."write", "values"=w226, "starting address"=w227) -> ("error out"=w224:errorcluster)  [unwired: 6 in, 2 out]
      }
      frame "停止命令" {
        n130 = call "CODCrMB_api.vi"("STEP"=enum16{"open", "read", "write", "close"}."write", "values"=u16[] [12], "starting address"=u16 4608) -> ("error out"=w250:errorcluster)  [unwired: 6 in, 2 out]
      }
      frame "量程切换" {
        n131 = case shown="\"H\"" w255 {
          tunnel: [u16[] [1] ("values") u16[] [0] ("values") _] -> w258
          frame "H" {
          }
          frame "L" {
          }
          frame "AUTO", Default {
          }
        }
        n132 = call "CODCrMB_api.vi"("STEP"=enum16{"open", "read", "write", "close"}."write", "values"=w258, "starting address"=u16 4276) -> ("error out"=w254:errorcluster)  [unwired: 6 in, 2 out]
      }
    }
  }
  n133 = while {
    stop <- FALSE stop-if-true
    # "测量数据、状态告警、关键参数解析显示"
    n134 = flat-sequence {
      frame #0 {
        n135 = global read "CODcr全局变量.vi" "测量数据区"() -> (w306:T4)
        "测量数据区" <- w306
        n136 = Unbundle By Name(w306) -> ("标样参考值"=→"标样参考值":sgl, "水样实测值"=w314:sgl, "标样实测值"=w312:sgl, "空白实测值"=w309:sgl, "零点核查实测值"=w311:sgl, "跨度核查实测值"=w310:sgl, "加标回收实测值"=w307:sgl, "平行样实测值"=w308:sgl)
        n137 = property on="工作状态" class="Enum (严格)"() -> ("RingText.Text"=w315:string)  [unwired: 2 in, 2 out]
        n138 = case shown="\"空白测试\"" w315 {
          tunnel: w314 -> [_ w318 _ _ _ _ _ _]
          tunnel: [w317 w318 w319 w320 w321 w322 w323 w324] -> w313
          tunnel: w312 -> [_ _ w319 _ _ _ _ _]
          tunnel: w311 -> [_ _ _ w320 _ _ _ _]
          tunnel: w310 -> [_ _ _ _ w321 _ _ _]
          tunnel: w309 -> [_ _ _ _ _ w322 _ _]
          tunnel: w308 -> [_ _ _ _ _ _ w323 _]
          tunnel: w307 -> [_ _ _ _ _ _ _ w324]
          frame "空闲", Default {
            n139 = local read "测量结果"() -> (w317:sgl)
          }
          frame "水样测试" {
          }
          frame "标样核查" {
          }
          frame "零点核查" {
          }
          frame "跨度核查" {
          }
          frame "空白测试" {
          }
          frame "平行样测试" {
          }
          frame "加标回收" {
          }
        }
        "测量结果" <- w313
      }
    }
    n140 = flat-sequence {
      frame #0 {
        n141 = global read "CODcr全局变量.vi" "状态告警区"() -> (w278:T3)
        "状态告警区" <- w278
        n142 = Unbundle By Name(w278) -> ("系统时间"=w290:timestamp, "工作状态"=w281:u16, "量程"=→"量程":u16)
        "仪器时间" <- w290
        "工作状态" <- w281
        n143 = Get Date/Time In Seconds() -> (seconds since 1Jan1904=w291:timestamp)
        "系统时间" <- w291
        n144 = Build Array(w291) -> (w285:timestamp[])
        n145 = Greater?(x=w281, y=T1."空闲") -> (0:w289:bool)
        n146 = Build Array(w290) -> (w284:timestamp[])
        n147 = global write "CODcr全局变量.vi" "工作状态"(w281) -> ()
        n148 = call "DateToHex.vi"("DATE"=w285) -> ("数组"=w282:u16[])  [unwired: 10 in]
        n149 = call "DateToHex.vi"("DATE"=w284) -> ("数组"=w283:u16[])  [unwired: 10 in]
        n150 = call <vilib>:"Boolean Crossing PtByPt.vi"("direction"=enum16{"either", "false-true", "true-false"}."false-true", "input"=w289) -> ("crossing"=w288:bool)  [unwired: 1 in]
        n151 = First Call?() -> (First Call?: T/F=w279:bool)
        n152 = Index Array(array=w282, index=2 ("索引")) -> (element=w293:u16)
        n153 = Or(x=w279, y=w288) -> (x .or. y?=w280:bool)
        n154 = Index Array(array=w283, index=2 ("索引")) -> (element=w294:u16)
        n155 = Split Number(x=w293) -> (hi(x)=w296:u8)  [unwired: 1 out]
        n156 = Split Number(x=w294) -> (hi(x)=w299:u8)  [unwired: 1 out]
        n157 = case shown="真" w280 {
          tunnel: w281 -> [_ w304]
          frame False {
          }
          frame True {
            n158 = Get Date/Time In Seconds() -> (seconds since 1Jan1904=→"启动时间":timestamp)
            "启动测量模式" <- w304
          }
        }
        n159 = To Byte Integer(number=w296) -> (8bit integer=w297:i8)
        n160 = To Byte Integer(number=w299) -> (8bit integer=w300:i8)
        n161 = Subtract(x=w300, y=w297) -> (x-y=w298:i8)
        n162 = Absolute Value(x=w298) -> (abs(x)=w301:i8)
        n163 = Greater Or Equal?(x=w301, y=i8 60) -> ()  [unwired: 1 out]
      }
    }
    n164 = global read "CODcr全局变量.vi" "定时控制"() -> (w262:T14)
    n165 = Wait (ms)(milliseconds to wait=u32 1000 ("等待时间（毫秒）")) -> ()  [unwired: 1 out]
    n166 = Unbundle By Name(w262) -> ("定时功能启用"=w261:bool)
    n167 = global read "CODcr全局变量.vi" "MB通信方式选择"() -> (w263:enum16{"串口", "TCP"})
    n168 = global read "CODcr全局变量.vi" "通讯状态"() -> (→"status":bool)
    n169 = local write "定时启动"(w261) -> ()
    n170 = local write "MB通信方式选择"(w263) -> ()
    n171 = case shown="\"TCP\"" w263 {
      tunnel: [w268 w269] -> w264
      frame "串口", Default {
        n172 = global read "CODcr全局变量.vi" "VISA Resource"() -> (w268:refnum<visa-resource-name>)
      }
      frame "TCP" {
        n173 = global read "CODcr全局变量.vi" "IP"() -> (w269:string)
      }
    }
    "COM口" <- w264
    n174 = flat-sequence {
      frame #0 {
        n175 = global read "CODcr全局变量.vi" "关键参数区"() -> (w270:T2)
        "关键参数区" <- w270
        n176 = Unbundle By Name(w270) -> ("测量精度"=→"测量精度":u16, "消解温度"=→"消解温度":u16, "消解时长"=→"消解时长":u16, "量程下限"=→"量程下限":sgl, "量程上限"=→"量程上限":sgl, "曲线斜率K"=→"曲线斜率K":sgl, "曲线斜率B"=→"曲线截距B":sgl)
      }
    }
  }
  n177 = while {
    tunnel: w6 -> [w326]
    tunnel: w5 -> [w325]
    stop <- FALSE stop-if-true
    n178 = event shown="[1] \"水样测试\": 值改变" {
      selector: _ -> [_ _ _ _ _ _ _ _ _ _ _ _ _ _ _ _ _ _ _ _ _ _ _ _]
      dyn-events: _ -> [_ _ _ _ _ _ _ _ _ _ _ _ _ _ _ _ _ _ _ _ _ _ _ _]
      timeout: _ -> [_ _ _ _ _ _ _ _ _ _ _ _ _ _ _ _ _ _ _ _ _ _ _ _]
      tunnel: w326 -> [_ _ _ _ _ _ _ _ _ _ _ _ _ _ _ w426 w445 _ _ _ w469 _ _ _]
      tunnel: w325 -> [_ _ _ _ _ _ _ _ _ _ _ _ _ _ _ w425 w444 _ _ _ w468 _ _ _]
      event Timeout {
        n179 = event-data() -> ()  [unwired: 1 in, 2 out]
      }
      event "水样测试": Value Change {
        n180 = event-data() -> ()  [unwired: 1 in, 6 out]
        n181 = local write "启动测量模式"(T1."水样测试" ("启动测量模式")) -> ()
        n182 = call "CODCrMB_api.vi"("STEP"=enum16{"open", "read", "write", "close"}."write", "values"=u16[] [1], "starting address"=u16 4608) -> ()  [unwired: 6 in, 3 out]
      }
      event "标样核查": Value Change {
        n183 = event-data() -> ()  [unwired: 1 in, 6 out]
        n184 = local write "启动测量模式"(T1."标样核查" ("启动测量模式")) -> ()
        n185 = call "CODCrMB_api.vi"("STEP"=enum16{"open", "read", "write", "close"}."write", "values"=u16[] [2], "starting address"=u16 4608) -> ()  [unwired: 6 in, 3 out]
      }
      event "零点核查": Value Change {
        n186 = event-data() -> ()  [unwired: 1 in, 6 out]
        n187 = local write "启动测量模式"(T1."零点核查" ("启动测量模式")) -> ()
        n188 = call "CODCrMB_api.vi"("STEP"=enum16{"open", "read", "write", "close"}."write", "values"=u16[] [3], "starting address"=u16 4608) -> ()  [unwired: 6 in, 3 out]
      }
      event "跨度核查": Value Change {
        n189 = event-data() -> ()  [unwired: 1 in, 6 out]
        n190 = local write "启动测量模式"(T1."跨度核查" ("启动测量模式")) -> ()
        n191 = call "CODCrMB_api.vi"("STEP"=enum16{"open", "read", "write", "close"}."write", "values"=u16[] [4], "starting address"=u16 4608) -> ()  [unwired: 6 in, 3 out]
      }
      event "空白测试": Value Change {
        n192 = event-data() -> ()  [unwired: 1 in, 6 out]
        n193 = local write "启动测量模式"(T1."空白测试" ("启动测量模式")) -> ()
        n194 = call "CODCrMB_api.vi"("STEP"=enum16{"open", "read", "write", "close"}."write", "values"=u16[] [5], "starting address"=u16 4608) -> ()  [unwired: 6 in, 3 out]
      }
      event "平行样测试": Value Change {
        n195 = event-data() -> ()  [unwired: 1 in, 6 out]
        n196 = local write "启动测量模式"(T1."平行样测试" ("启动测量模式")) -> ()
        n197 = call "CODCrMB_api.vi"("STEP"=enum16{"open", "read", "write", "close"}."write", "values"=u16[] [6], "starting address"=u16 4608) -> ()  [unwired: 6 in, 3 out]
      }
      event "加标回收测试": Value Change {
        n198 = event-data() -> ()  [unwired: 1 in, 6 out]
        n199 = local write "启动测量模式"(T1."加标回收" ("启动测量模式")) -> ()
        n200 = call "CODCrMB_api.vi"("STEP"=enum16{"open", "read", "write", "close"}."write", "values"=u16[] [7], "starting address"=u16 4608) -> ()  [unwired: 6 in, 3 out]
      }
      event "空白校准": Value Change {
        n201 = event-data() -> ()  [unwired: 1 in, 6 out]
        n202 = local write "启动测量模式"(T1."空白校准" ("启动测量模式")) -> ()
        n203 = call "CODCrMB_api.vi"("STEP"=enum16{"open", "read", "write", "close"}."write", "values"=u16[] [8], "starting address"=u16 4608) -> ()  [unwired: 6 in, 3 out]
      }
      event "标样校准": Value Change {
        n204 = event-data() -> ()  [unwired: 1 in, 6 out]
        n205 = local write "启动测量模式"(T1."标样校准" ("启动测量模式")) -> ()
        n206 = call "CODCrMB_api.vi"("STEP"=enum16{"open", "read", "write", "close"}."write", "values"=u16[] [9], "starting address"=u16 4608) -> ()  [unwired: 6 in, 3 out]
      }
      event "停止": Value Change {
        n207 = event-data() -> ()  [unwired: 1 in, 6 out]
        n208 = Two Button Dialog(message="确认是否停止？" ("消息"), 1:"否" ("F按钮名称（“取消”）"), 2:"是" ("T按钮名称（“确定”）")) -> (T button?=w364:bool)
        n209 = case shown="真" w364 {
          frame False {
          }
          frame True {
            n210 = Obtain Notifier(name (unnamed)="CODCr" ("名称（未命名）"), notification data type=FALSE) -> (notifier out=w372:refnum<notifier>, error out=w370:errorcluster)  [unwired: 2 in, 1 out]
            n211 = call "CODCrMB_api.vi"("STEP"=enum16{"open", "read", "write", "close"}."write", "values"=u16[] [12], "starting address"=u16 4608) -> ()  [unwired: 6 in, 3 out]
            n212 = Send Notification(notification=TRUE ("通知"), notifier=w372, error in (no error)=w370) -> (notifier out=w369:refnum<notifier>, error out=w368:errorcluster)
            n213 = Release Notifier(notifier=w369, error in (no error)=w368) -> ()  [unwired: 1 in, 3 out]
          }
        }
      }
      event "保存KB值": Value Change {
        n214 = event-data() -> ()  [unwired: 1 in, 6 out]
        n215 = local read "曲线截距B"() -> (w378:sgl)
        n216 = local read "曲线斜率K"() -> (w379:sgl)
        n217 = Build Array(w379, w378) -> (w384:sgl[])
        n218 = call "FloatToHex.vi"("浮点数"=w384) -> ("DCBA整形输出"=w381:u16[])  [unwired: 10 in]
        n219 = call "CODCrMB_api.vi"("STEP"=enum16{"open", "read", "write", "close"}."write", "values"=w381, "starting address"=u16 4263) -> ("error out"=w380:errorcluster)  [unwired: 6 in, 2 out]
        n220 = case shown="无错误" w380 {
          tunnel: w379 -> [w386 _]
          tunnel: w378 -> [w385 _]
          frame No Error {
            n221 = global read "CODcr全局变量.vi" "CODCr仪器参数"() -> (w388:T15)
            n222 = Bundle By Name(cluster=w388, "曲线截距"=w385, "曲线斜率"=w386) -> (w387:T15)
            n223 = global write "CODcr全局变量.vi" "CODCr仪器参数"(w387) -> ()
          }
          frame Error {
          }
        }
      }
      event "定时启动": Value Change {
        n224 = event-data() -> ()  [unwired: 1 in, 6 out]
        n225 = flat-sequence {
          frame #0 {
            n226 = global read "CODcr全局变量.vi" "定时控制"() -> (w390:T14)
            n227 = call "周期设置.vi"("定时控制输入"=w390) -> ("定时控制输出"=w389:T16)  [unwired: 10 in]
            n228 = global write "CODcr全局变量.vi" "定时控制"(w389) -> ()
          }
          frame #1 {
            n229 = call "配置文件保存.vi"() -> ()  [unwired: 12 in]
          }
        }
      }
      event "仪器参数": Value Change {
        n230 = event-data() -> ()  [unwired: 1 in, 6 out]
        n231 = global read "CODcr全局变量.vi" "CODCr仪器参数"() -> (w392:T15)
        n232 = call "仪器参数设置.vi"("氨氮仪器参数"=w392) -> ("仪器参数设置输出"=w391:T17)  [unwired: 10 in]
        n233 = Unbundle By Name(w391) -> ("确定"=w393:bool)
        n234 = case shown="真" w393 {
          tunnel: w392 -> [_ w395]
          tunnel: w391 -> [_ w394]
          frame False {
          }
          frame True {
            n235 = flat-sequence {
              tunnel: w395 -> [w412]
              tunnel: w394 -> [w411]
              frame #0 {
                n236 = Unbundle By Name(w411) -> ("测量量程"=w410:dbl, "测量精度"=w409:dbl, "测量间隔"=w408:dbl, "消解温度"=w407:dbl, "消解时长"=w406:dbl, "空白校准时间"=w405:timestamp, "曲线截距"=w404:dbl, "曲线斜率"=w403:dbl, "测量检出限"=w402:dbl, "测量信号值"=w401:dbl, "线性相关系数"=w400:dbl, "二次多项式系数"=w399:dbl, "标样校准时间"=w398:timestamp, "稀释倍数"=w397:dbl)
                n237 = Bundle By Name(cluster=w412, "测量量程"=w410, "测量精度"=w409, "测量间隔"=w408, "消解温度"=w407, "消解时长"=w406, "空白校准时间"=w405, "曲线截距"=w404, "曲线斜率"=w403, "测量检出限"=w402, "测量信号值"=w401, "线性相关系数"=w400, "二次多项式系数"=w399, "标样校准时间"=w398, "稀释倍数"=w397) -> (w396:T15)
                n238 = global write "CODcr全局变量.vi" "CODCr仪器参数"(w396) -> ()
              }
              frame #1 {
                n239 = call "配置文件保存.vi"() -> ()  [unwired: 12 in]
              }
            }
          }
        }
      }
      event "质控参数": Value Change {
        n240 = event-data() -> ()  [unwired: 1 in, 6 out]
        n241 = global read "CODcr全局变量.vi" "质控参数设置"() -> (w414:T18)
        n242 = call "质控参数设置.vi"("质控参数设置"=w414) -> ("输出簇"=w413:T19)  [unwired: 10 in]
        n243 = Unbundle By Name(w413) -> ("确定"=w415:bool)
        n244 = case shown="真" w415 {
          tunnel: w414 -> [_ w417]
          tunnel: w413 -> [_ w416]
          frame False {
          }
          frame True {
            n245 = flat-sequence {
              tunnel: w417 -> [w424]
              tunnel: w416 -> [w423]
              frame #0 {
                n246 = Unbundle By Name(w423) -> ("跨度值"=w421:dbl, "零点标准液浓度"=w420:dbl, "跨度标准液浓度"=w419:dbl, "标准液标准浓度"=w418:dbl)
                n247 = Bundle By Name(cluster=w424, "跨度值"=w421, "零点标准液浓度"=w420, "跨度标准液浓度"=w419, "标准液标准浓度"=w418) -> (w422:T18)
                n248 = global write "CODcr全局变量.vi" "质控参数设置"(w422) -> ()
              }
              frame #1 {
                n249 = call "配置文件保存.vi"() -> ()  [unwired: 12 in]
              }
            }
          }
        }
      }
      event "打开串口": Value Change {
        n250 = event-data() -> ()  [unwired: 1 in, 6 out]
        n251 = flat-sequence {
          tunnel: w426 -> [w428]
          tunnel: w425 -> [w427]
          frame #0 {
            n252 = global read "CODcr全局变量.vi" "VISA Resource"() -> (w435:refnum<visa-resource-name>)
            n253 = global read "CODcr全局变量.vi" "PORT"() -> (w429:string)
            n254 = global read "CODcr全局变量.vi" "IP"() -> (w430:string)
            n255 = call "串口配置.vi"("PORT"=w429, "IP"=w430, "请选择串口:"=w435) -> ("PORT 2"=w431:string, "IP 2"=w432:string, "确认 2"=w434:bool, "VISA资源名称 2"=w433:refnum<visa-resource-name>)  [unwired: 5 in]
            n256 = case shown="真" w434 {
              tunnel: w433 -> [_ w438]
              tunnel: w428 -> [_ w440]
              tunnel: w427 -> [_ w439]
              tunnel: w432 -> [_ w437]
              tunnel: w431 -> [_ w436]
              frame False {
              }
              frame True {
                n257 = global write "CODcr全局变量.vi" "VISA Resource"(w438) -> ()
                n258 = global write "CODcr全局变量.vi" "PORT"(w436) -> ()
                n259 = global write "CODcr全局变量.vi" "IP"(w437) -> ()
                n260 = Bundle By Name(cluster=cluster{"命令":string} {"命令"=""} ("元素"), "命令"="启用模块" ("名称（未命名）")) -> (w441:cluster{"命令":string})
                n261 = Enqueue Element(queue=w440, element=w441, error in (no error)=w439) -> ()  [unwired: 1 in, 3 out]
              }
            }
          }
          frame #1 {
            n262 = call "配置文件保存.vi"() -> ()  [unwired: 12 in]
          }
        }
      }
      event "释放串口": Value Change {
        n263 = event-data() -> ()  [unwired: 1 in, 6 out]
        n264 = Two Button Dialog(message="确认是否释放串口，释放串口将导致通信失败！" ("消息")) -> (T button?=w446:bool)  [unwired: 2 in]
        n265 = case shown="真" w446 {
          tunnel: w445 -> [_ w449]
          tunnel: w444 -> [_ w448]
          frame False {
          }
          frame True {
            n266 = Bundle By Name(cluster=cluster{"命令":string} {"命令"=""} ("元素"), "命令"="停用模块" ("名称（未命名）")) -> (w450:cluster{"命令":string})
            n267 = Enqueue Element(queue=w449, element=w450, error in (no error)=w448) -> ()  [unwired: 1 in, 3 out]
          }
        }
      }
      event "MB通信方式选择": Value Change {
        n268 = event-data() -> ()  [unwired: 1 in, 6 out]
        n269 = flat-sequence {
          frame #0 {
            n270 = global write "CODcr全局变量.vi" "MB通信方式选择"("MB通信方式选择") -> ()
          }
          frame #1 {
            n271 = call "配置文件保存.vi"() -> ()  [unwired: 12 in]
          }
        }
      }
      event "写入消解温度时长": Value Change {
        n272 = event-data() -> ()  [unwired: 1 in, 6 out]
        n273 = local read "消解时长"() -> (w458:u16)
        n274 = local read "消解温度"() -> (w459:u16)
        n275 = Build Array(w459, w458) -> (w457:u16[])
        n276 = call "WordToHex.vi"("WORD"=w457) -> ("数组"=w454:u16[])  [unwired: 10 in]
        n277 = call "CODCrMB_api.vi"("STEP"=enum16{"open", "read", "write", "close"}."write", "values"=w454, "starting address"=u16 4257) -> ()  [unwired: 6 in, 3 out]
      }
      event "校时": Value Change {
        n278 = event-data() -> ()  [unwired: 1 in, 6 out]
        n279 = Get Date/Time In Seconds() -> (seconds since 1Jan1904=w467:timestamp)
        n280 = Build Array(w467) -> (w464:timestamp[])
        n281 = call "DateToHex.vi"("DATE"=w464) -> ("数组"=w463:u16[])  [unwired: 10 in]
        n282 = Insert Into Array(array=u16[] [13] ("values"), index=1 ("索引"), new element=w463) -> (w460:u16[])
        n283 = call "CODCrMB_api.vi"("STEP"=enum16{"open", "read", "write", "close"}."write", "values"=w460, "starting address"=u16 4608) -> ()  [unwired: 6 in, 3 out]
      }
      event "设置": Value Change {
        n284 = event-data() -> ()  [unwired: 1 in, 6 out]
        n285 = property on="窗格" class="Pane"("Origin"=T6 {"Horizontal"=0, "Vertical"=728} ("原点")) -> ()  [unwired: 2 in, 2 out]
        n286 = Bundle By Name(cluster=cluster{"命令":string} {"命令"=""} ("元素"), "命令"="CODCr读取参数" ("名称（未命名）")) -> (w470:cluster{"命令":string})
        n287 = Enqueue Element(queue=w469, element=w470, error in (no error)=w468) -> ()  [unwired: 1 in, 3 out]
      }
      event "返回": Value Change {
        w474 = FALSE ("可见")
        n288 = event-data() -> ()  [unwired: 1 in, 6 out]
        n289 = property on="窗格" class="Pane"("Origin"=T6 {"Horizontal"=0, "Vertical"=0} ("原点")) -> ()  [unwired: 2 in, 2 out]
        n290 = property on="写入消解温度时长" class="Bool"("Visible"=w474) -> ()  [unwired: 2 in, 2 out]
        n291 = property on="释放串口" class="Bool"("Visible"=w474) -> ()  [unwired: 2 in, 2 out]
        n292 = property on="打开串口" class="Bool"("Visible"=w474) -> ()  [unwired: 2 in, 2 out]
        n293 = property on="MB通信方式选择" class="Enum (严格)"("Visible"=w474) -> ()  [unwired: 2 in, 2 out]
      }
      event "曲线斜率K", "曲线截距B", "消解温度", "消解时长": Mouse Down {
        n294 = event-data() -> ("CtlRef"=w478:refnum<vi>)  [unwired: 1 in, 7 out]
        n295 = property class="DigNum"(reference=w478) -> (reference out=w479:refnum<vi>, "Value"=w477:variant)  [unwired: 1 in, 1 out]
        n296 = Variant To Data(Variant=w477) -> (data=w476:sgl)  [unwired: 2 in, 1 out]
        n297 = call "CODCR数字键盘.vi"("OldNumber"=w476) -> ("NewNumber"=w480:sgl)
        n298 = property class="DigNum"(reference=w479, "Value"=w480) -> ()  [unwired: 1 in, 2 out]
      }
      event "隐藏按钮": Value Change {
        n299 = event-data() -> ("NewVal"=w481:bool)  [unwired: 1 in, 5 out]
        n300 = property on="写入消解温度时长" class="Bool"("Visible"=w481) -> ()  [unwired: 2 in, 2 out]
        n301 = property on="释放串口" class="Bool"("Visible"=w481) -> ()  [unwired: 2 in, 2 out]
        n302 = property on="打开串口" class="Bool"("Visible"=w481) -> ()  [unwired: 2 in, 2 out]
        n303 = property on="MB通信方式选择" class="Enum (严格)"("Visible"=w481) -> ()  [unwired: 2 in, 2 out]
      }
    }
  }
  n304 = while {
    tunnel: w6 -> [w483]
    tunnel: w5 -> [w482]
    i -> [w491]
    stop <- FALSE stop-if-true
    n305 = First Call?() -> (First Call?: T/F=w486:bool)
    n306 = case shown="真" w486 {
      tunnel: w483 -> [w495 w500]
      tunnel: w482 -> [w494 w499]
      tunnel: [w495 w498] -> w485
      tunnel: [w494 w497] -> w484
      frame False {
      }
      frame True {
        n307 = Bundle By Name(cluster=cluster{"命令":string} {"命令"=""} ("元素"), "命令"="CODMn读取参数" ("名称（未命名）")) -> (w503:cluster{"命令":string})
        n308 = Enqueue Element(queue=w500, element=w503, timeout in ms (-1)=1000 ("超时毫秒(-1)"), error in (no error)=w499) -> (queue out=w498:refnum<queue>, error out=w497:errorcluster)  [unwired: 1 out]
      }
    }
    n309 = Get Queue Status(queue=w485, error in (no error)=w484) -> (queue out=w489:refnum<queue>, error out=w488:errorcluster, # elements in queue=w490:i32)  [unwired: 1 in, 5 out]
    n310 = Equal To 0?(x=w490) -> (x = 0?=w487:bool)
    n311 = case shown="真" w487 {
      tunnel: w489 -> [_ w505]
      tunnel: w488 -> [_ w504]
      frame False {
      }
      frame True {
        n312 = Bundle By Name(cluster=cluster{"命令":string} {"命令"=""} ("元素"), "命令"="CODCr读取" ("名称（未命名）")) -> (w507:cluster{"命令":string})
        n313 = Enqueue Element(queue=w505, element=w507, timeout in ms (-1)=1000 ("超时毫秒(-1)"), error in (no error)=w504) -> ()  [unwired: 3 out]
      }
    }
    n314 = Wait (ms)(milliseconds to wait=u32 1000 ("等待时间（毫秒）")) -> ()  [unwired: 1 out]
    "主循环次数" <- w491
  }
